vi "Move Right To Matrix.vi"(3 "Make Vertical":bool, 5 "Label":string="Test", 6 "Wait Time":dbl, 8 "error in":errorcluster, 9 "Speed (mm/s)":dbl=50.0, 10 "Goal Pose in Location":T1 format="%.3f", 11 "Location":string="Base") -> (0 "error out":errorcluster)   [LabVIEW 2013]
uses:
  <vilib>/Analysis/Matrix/Datatypes/RealMatrix.ctl
  <vilib>/Analysis/Matrix/NI_Matrix.lvlib
panel:
  out "Start Pose":T1
  out "step":i32
  out "Int Pose":T1 format="%.3f"
  out "End Pose":T1 format="%.3f"
  in  "Alt Goal":T2
  in  "Start":T1 format="%.3f"
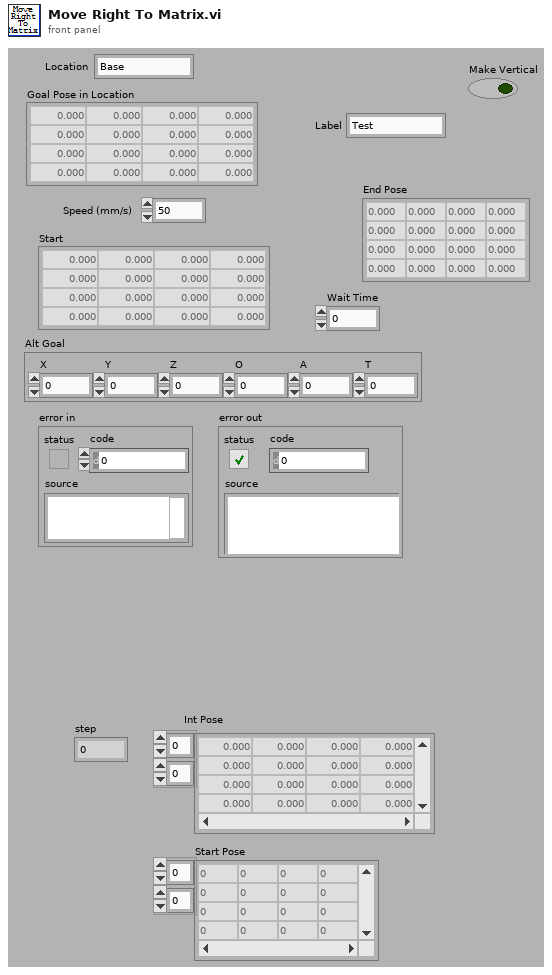
[diagram p1: front panel]
types:
  T1 = typedef "NI_Matrix.lvlib/RealMatrix.ctl" = dbl[][]
  T2 = cluster{"X":dbl, "Y":dbl, "Z":dbl, "O":dbl, "A":dbl, "T":dbl}
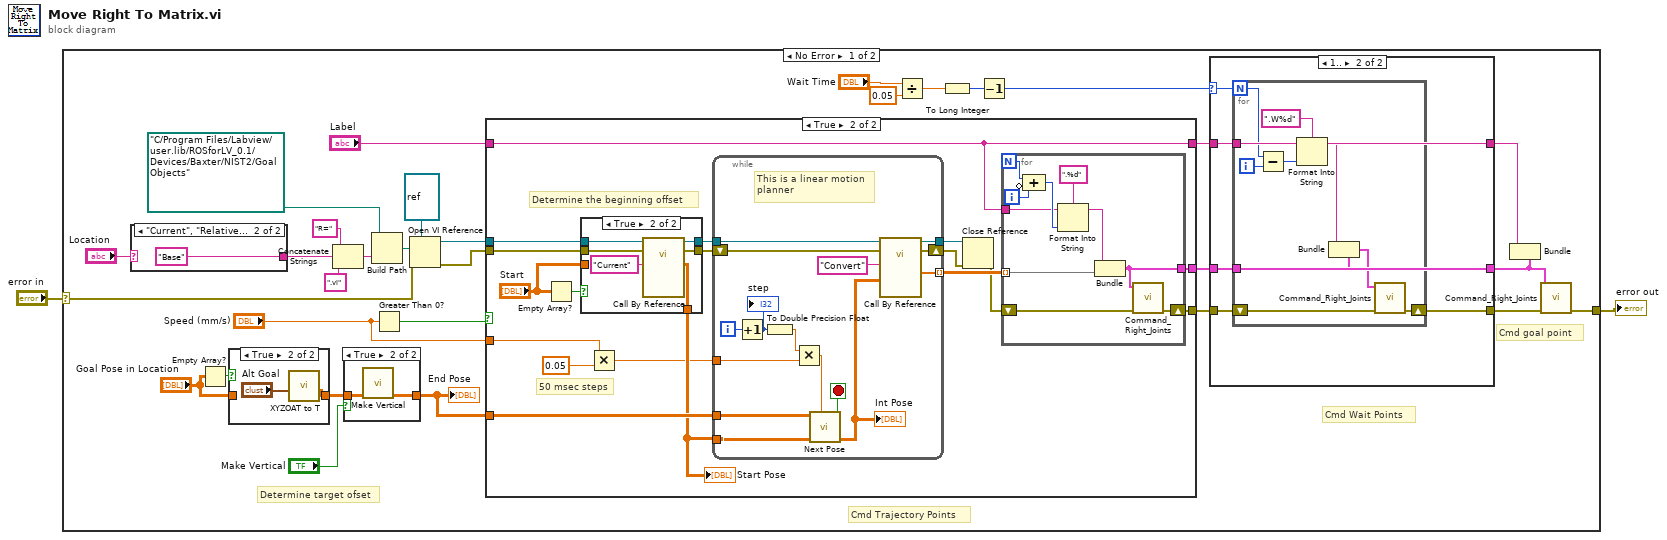
[diagram p0: block diagram]
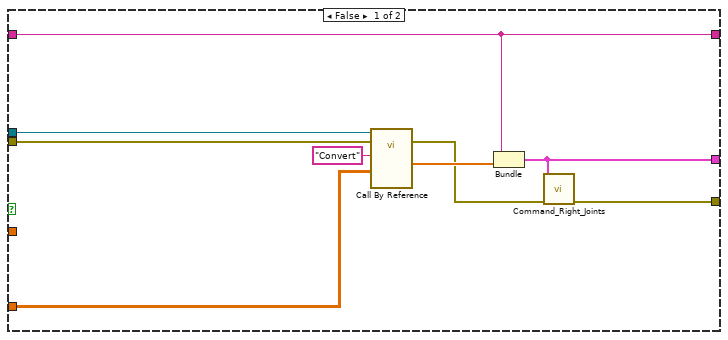
[diagram p5: hidden frame]
diagram:
  n1 = case shown="No Error" "error in" {
    selector: "error in" -> [w13 w121]
    tunnel: [w6 w121] -> w1
    frame No Error {
      # "Determine target ofset"
      # "Cmd goal point"
      # "Cmd Wait Points"
      # "Cmd Trajectory Points"
      n2 = case shown="\"Current\", \"Relative\"" "Location" {
        selector: "Location" -> [w34 _]
        tunnel: [w34 "Base"] -> w14
        frame Default {
        }
        frame "Current", "Relative" {
        }
      }
      n3 = Empty Array?(array="Goal Pose in Location") -> (empty?=w33:bool)
      n4 = case shown="True" w33 {
        tunnel: "Goal Pose in Location" -> [w118 _]
        tunnel: [w118 w119] -> w29
        frame False {
        }
        frame True {
          n5 = call "XYZOAT to T.vi"("XYZOAT"="Alt Goal") -> ("T"=w119:T1)  [unwired: 10 in]
        }
      }
      n6 = Concatenate Strings("R=", w14, ".vi" ("string")) -> (w19:string)
      n7 = case shown="True" "Make Vertical" {
        tunnel: w29 -> [w54 w56]
        tunnel: [w54 w55] -> w28
        frame False {
        }
        frame True {
          n8 = call "Make Vertical.vi"("Matrix"=w56) -> ("Vertical Matrix"=w55:T1)  [unwired: 10 in]
        }
      }
      "End Pose" <- w28
      n9 = Build Path(base path=path "C:/Program Files/Labview/user.lib/ROSforLV_0.1/Devices/Baxter/NIST2/Goal Objects", name or relative path=w19) -> (appended path=w20:path)
      n10 = Greater Than 0?(x="Speed (mm/s)") -> (x > 0?=w32:bool)
      n11 = Open VI Reference(type specifier VI Refnum (for type only)=refnum<vi> refnum, vi path=w20, error in (no error)=w13) -> (vi reference=w5:refnum<vi>, error out=w4:errorcluster)  [unwired: 3 in]
      n12 = case shown="True" w32 {
        tunnel: "Label" -> [w57 w79]
        tunnel: w28 -> [w62 w83]
        tunnel: "Speed (mm/s)" -> [_ w66]
        tunnel: w5 -> [w64 w72]
        tunnel: w4 -> [w63 w71]
        tunnel: [w60 w81] -> w12
        tunnel: [w58 w80] -> w10
        tunnel: [w57 w79] -> w11
        frame False {
          n13 = call-by-ref "?"(reference=w64, error in=w63, "Matrix"=w62, "Command"="Convert") -> (error out=w59:errorcluster, "Joints"=w61:dbl[])  [unwired: 7 in, 3 out]
          n14 = Bundle("Label"=w57, "Joints"=w61) -> (w60:cluster{"Label":string, "Joints":dbl[]})  [unwired: 1 in]
          n15 = call "Command_Right_Joints.vi"("error in"=w59, "Goal"=w60) -> ("error out"=w58:errorcluster)  [unwired: 6 in, 1 out]
        }
        frame True {
          # "50 msec steps"
          # "Determine the beginning offset"
          n16 = Empty Array?(array="Start") -> (empty?=w69:bool)
          n17 = case shown="True" w69 {
            tunnel: [w84 w92] -> w73
            tunnel: w71 -> [w84 w91]
            tunnel: [w85 w90] -> w74
            tunnel: w72 -> [w85 w88]
            tunnel: "Start" -> [w86 _]
            tunnel: [w86 w87] -> w75
            frame False {
            }
            frame True {
              n18 = call-by-ref "?"(reference=w88, error in=w91, "Command"="Current") -> (reference out=w90:refnum<vi>, error out=w92:errorcluster, "Matrix"=w87:T1)  [unwired: 8 in, 2 out]
            }
          }
          "Start Pose" <- w75
          n19 = Multiply(x=w66, y=0.05) -> (x*y=w67:dbl)
          n20 = while {
            tunnel: w75 -> [w114]
            tunnel: w83 -> [w113]
            tunnel: w74 -> [w110]
            tunnel: [w107] -> w82 mode=indexing
            shift-right: [w106] -> w77
            shift-left: w73 -> [w109]
            tunnel: [w105] -> w78
            tunnel: w67 -> [w104]
            i -> [w116]
            stop <- w117 stop-if-true
            # "This is a linear motion\nplanner"
            n21 = Increment(x=w116) -> (x+1=w112:i32)
            "step" <- w112
            n22 = To Double Precision Float(number=w112) -> (double precision float=w103:dbl)
            n23 = Multiply(x=w103, y=w104) -> (x*y=w115:dbl)
            n24 = call "Next Pose.vi"("Step"=w115, "Start"=w114, "Goal"=w113) -> ("Pose"=w108:T1, "At Goal"=w117:bool)  [unwired: 7 in]
            "Int Pose" <- w108
            n25 = call-by-ref "Call By Reference"(reference=w110, error in=w109, "Matrix"=w108, "Command"="Convert") -> (reference out=w105:refnum<vi>, error out=w106:errorcluster, "Joints"=w107:dbl[])  [unwired: 7 in, 2 out]
          }
          n26 = Close Reference(reference=w78, error in (no error)=w77) -> (error out=w76:errorcluster)
          n27 = for {
            N -> [w102]
            tunnel: w79 -> [w98]
            tunnel: w82 -> [w96] mode=indexing
            shift-right: [w94] -> w80
            shift-left: w76 -> [w95]
            tunnel: [w93] -> w81
            i -> [w101]
            n28 = Compound Arithmetic op=ADD(w102, invert w101) -> (w99:i32)
            n29 = Format Into String(format string=".%d", initial string=w98, w99) -> (resulting string=w97:string)  [unwired: 1 in, 1 out]
            n30 = Bundle(w97, "Joints"=w96) -> (w93:cluster{string, "Joints":dbl[]})  [unwired: 1 in]
            n31 = call "Command_Right_Joints.vi"("error in"=w95, "Goal"=w93) -> ("error out"=w94:errorcluster)  [unwired: 6 in, 1 out]
          }
        }
      }
      n32 = Divide(x="Wait Time", y=0.05) -> (x/y=w23:dbl)
      n33 = To Long Integer(number=w23) -> (32bit integer=w22:i32)
      n34 = Decrement(x=w22) -> (x-1=w24:i32)
      n35 = case shown="1.." w24 {
        selector: w24 -> [_ w43]
        tunnel: w12 -> [w37 w40]
        tunnel: w11 -> [w36 w39]
        tunnel: w10 -> [w38 w42]
        tunnel: [w38 w41] -> w9
        tunnel: [w37 w40] -> w8
        tunnel: [w36 w39] -> w7
        frame ..0 {
        }
        frame 1.. {
          n36 = for {
            N: w43 -> [w52]
            tunnel: w39 -> [w44]
            tunnel: w40 -> [w49]
            shift-right: [w45] -> w41
            shift-left: w42 -> [w46]
            i -> [w51]
            n37 = Subtract(x=w52, y=w51) -> (x-y=w53:i32)
            n38 = Format Into String(format string=".W%d", initial string=w44, w53) -> (resulting string=w48:string)  [unwired: 1 in, 1 out]
            n39 = Bundle(cluster=w49, "Label"=w48) -> (w47:cluster{"Label":string, "Joints":dbl[]})  [unwired: 1 in]
            n40 = call "Command_Right_Joints.vi"("error in"=w46, "Goal"=w47) -> ("error out"=w45:errorcluster)  [unwired: 6 in, 1 out]
          }
        }
      }
      n41 = Bundle(cluster=w8, "Label"=w7) -> ()  [unwired: 1 in, 1 out]
      n42 = call "Command_Right_Joints.vi"("error in"=w9, "Goal"=w8) -> ("error out"=w6:errorcluster)  [unwired: 6 in, 1 out]
    }
    frame Error {
    }
  }
  "error out" <- w1
